vi "ReplaceSelf.vi"(0 "XRef":T13, 1 "Terms":T10, 2 "Diagram":T9, 3 "State In":T4 {"BlockNodeState"."Draw Style" items=["FunctionBlock", "ExpressVI", "Variable", "Elemental I/O", "32x32 Icon", "FunctionBlockCompact"]; "BlockNodeState"."Terminal Data"."Terminal Flags" format="%.0b"}) -> (14 "Replace Self?":T3, 15 "Reply":T1)   [LabVIEW 2018, in "N9010A_SCPI Node.xnode"]
uses:
  N9010A_SCPI Node.xnode
  <vilib>/XNodeSupport/XNodeXNodeRef.ctl
  <vilib>/XNodeSupport/XNodeTermIDPairs.ctl
  <vilib>/XNodeSupport/XNodeTermIDPair.ctl
  <vilib>/XNodeSupport/XNodeTermRef.ctl
  <vilib>/XNodeSupport/XNodeString.ctl
  <vilib>/XNodeSupport/XNodeTopLevelDiagramRef.ctl
  State.ctl
  <vilib>/BlockNodeSupport/BlockNodeState.ctl
  <vilib>/BlockNodeSupport/TerminalData.ctl
  <vilib>/picture/picture.llb/imagedata.ctl
  Utility/command_spec.ctl
  <vilib>/XNodeSupport/XNodeBool.ctl
  <vilib>/XNodeSupport/XNodeStringArray.ctl
  <vilib>/Utility/miscctls.llb/LVPointTypeDef.ctl
  <vilib>/XNodeSupport/NI_XNodeSupport.lvlib
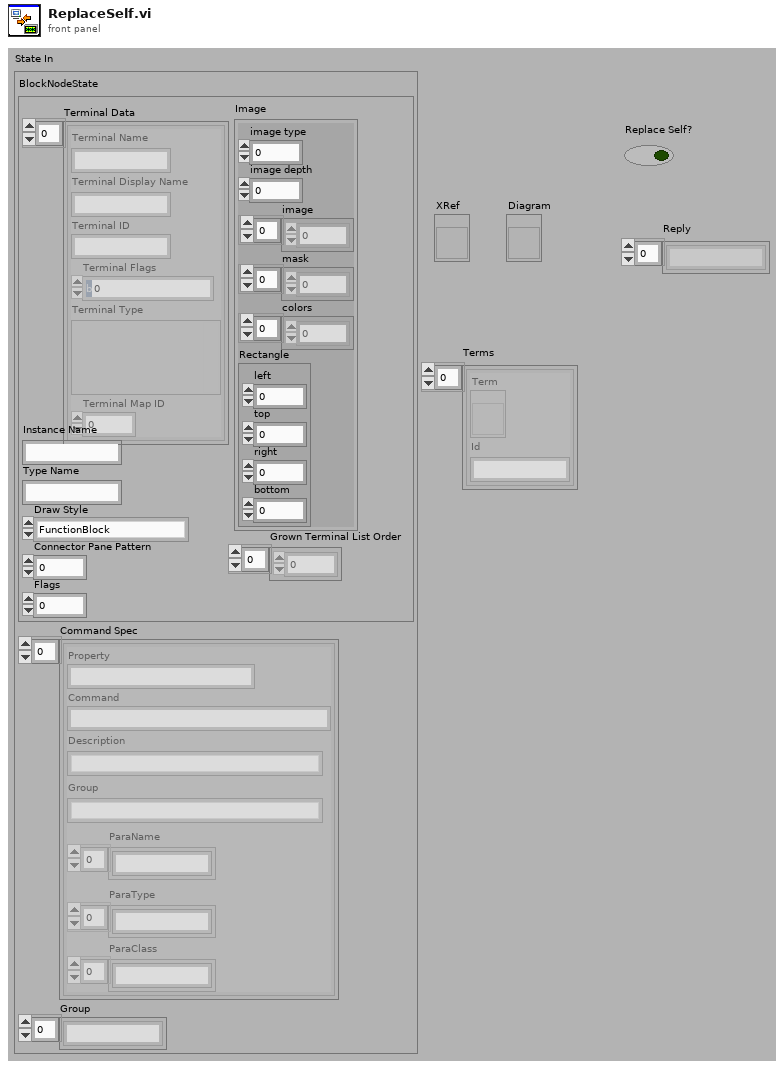
[diagram p1: front panel]
types:
  T1 = typedef "NI_XNodeSupport.lvlib/XNodeStringArray.ctl" = T2[]
  T2 = typedef "NI_XNodeSupport.lvlib/XNodeString.ctl" = string
  T3 = typedef "NI_XNodeSupport.lvlib/XNodeBool.ctl" = bool
  T4 = typedef "N9010A_SCPI Node.xnode/State.ctl" = cluster{"BlockNodeState":T5, "Command Spec":T8, "Group":string[]}
  T5 = typedef "BlockNodeState.ctl" = cluster{"Terminal Data":T6[], "Instance Name":string, "Type Name":string, "Draw Style":i32, "Connector Pane Pattern":i32, "Flags":i32, "Grown Terminal List Order":i32[], "Image":T7}
  T6 = typedef "TerminalData.ctl" = cluster{"Terminal Name":string, "Terminal Display Name":string, "Terminal ID":string, "Terminal Flags":i32, "Terminal Type":variant, "Terminal Map ID":i32}
  T7 = typedef "imagedata.ctl" = cluster{"image type":i32, "image depth":i32, "image":u8[], "mask":u8[], "colors":u32[], "Rectangle":cluster{"left":i16, "top":i16, "right":i16, "bottom":i16}}
  T8 = typedef "command_spec.ctl" = cluster{"Property":string, "Command":string, "Description":string, "Group":string, "ParaName":string[], "ParaType":string[], "ParaClass":string[]}[]
  T9 = typedef "NI_XNodeSupport.lvlib/XNodeTopLevelDiagramRef.ctl" = refnum<vi>
  T10 = typedef "NI_XNodeSupport.lvlib/XNodeTermIDPairs.ctl" = T11[]
  T11 = typedef "NI_XNodeSupport.lvlib/XNodeTermIDPair.ctl" = cluster{"Term":T12, "Id":T2}
  T12 = typedef "NI_XNodeSupport.lvlib/XNodeTermRef.ctl" = refnum<vi>
  T13 = typedef "NI_XNodeSupport.lvlib/XNodeXNodeRef.ctl" = refnum<vi>
  T14 = typedef "LVPointTypeDef.ctl" = cluster{"Horizontal":i16, "Vertical":i16}
  T15 = cluster{"Property":string, "Command":string, "Description":string, "Group":string, "ParaName":string[], "ParaType":string[], "ParaClass":string[]}
  T16 = typedef "LVRectTypeDef.ctl" = cluster{"Left":i16, "Top":i16, "Right":i16, "Bottom":i16}
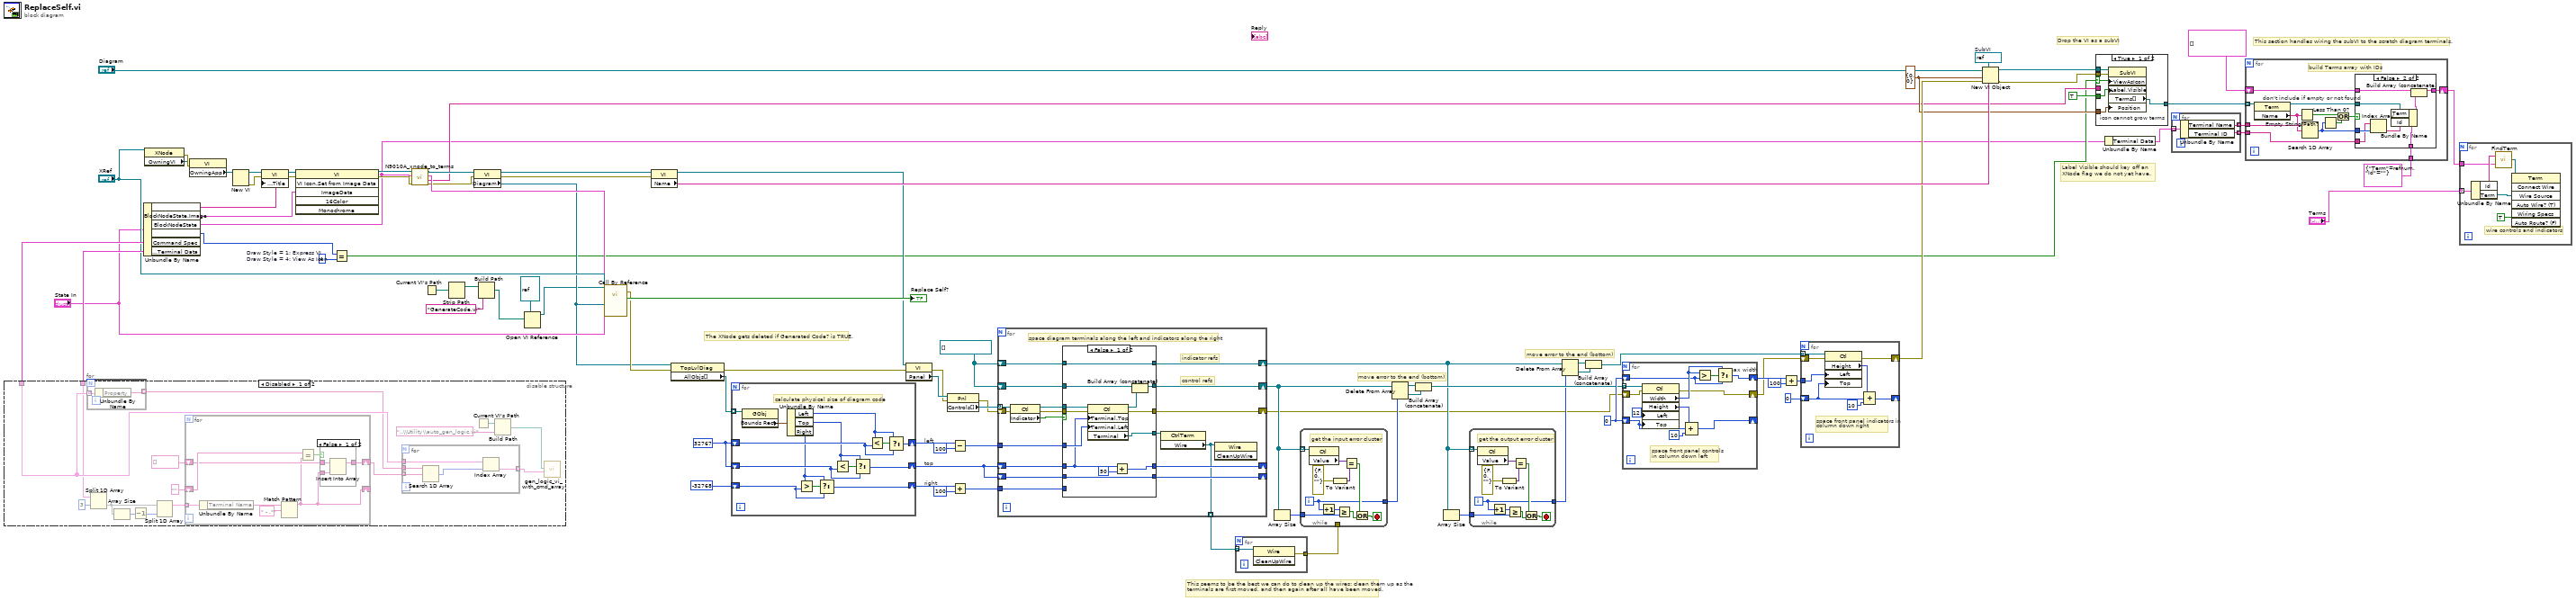
[diagram p0: block diagram]
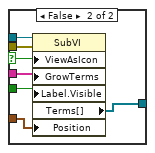
[diagram p2: hidden frame]
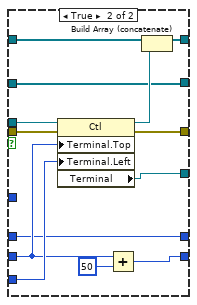
[diagram p4: hidden frame]
diagram:
  w6 = 4  # Draw Style = 1: Express VI Draw Style = 4: View As Icon
  w45 = 0 ("Position:Left")
  w46 = refnum<vi>[] []
  w60 = i16 32767 ("left")
  w8 = T14 {"Horizontal"=0, "Vertical"=0} ("location")
  w79 = refnum<vi> refnum  # SubVI
  # "Label Visible should key off an XNode flag we do not yet have."
  # "Drop the VI as a subVI"
  # "This section handles wiring the subVI to the scratch diagram terminals."
  # "The XNode gets deleted if Generated Code? is TRUE."
  # "This seems to be the best we can do to clean up the wires: clean them up as the terminals are first moved, and then again after all have been moved."
  # "move error to the end (bottom)"
  # "move error to the end (bottom)"
  # "right"
  # "top"
  # "left"
  n1 = Unbundle By Name("State In") -> ("BlockNodeState.Type Name"=w83:string, "BlockNodeState.Image"=w82:T7, "BlockNodeState"=w2:T5, "BlockNodeState.Draw Style"=w5:i32, "Command Spec"=w77:T8, "BlockNodeState.Terminal Data"=w76:T6[])
  n2 = disable-structure shown="Disabled" {
    disable-tunnel: w77 -> [w103 _]
    disable-tunnel: w76 -> [w102 _]
    frame Disabled {
      n3 = for {
        tunnel: [w121] -> _ mode=indexing
        tunnel: [w122] -> w93 mode=indexing
        tunnel: w103 -> [w121] mode=indexing
        n4 = Unbundle By Name(w121) -> ("Property"=w122:string)
      }
      n5 = Split 1D Array(array=w102, index=3) -> (second subarray=w98:T6[])  [unwired: 1 out]
      n6 = Array Size(array=w98) -> (size(s)=w100:i32)
      n7 = Decrement(x=w100) -> (x-1=w99:i32)
      n8 = Split 1D Array(array=w98, index=w99) -> (first subarray=w97:T6[])  [unwired: 1 out]
      n9 = for {
        tunnel: w97 -> [w116] mode=indexing
        shift-right: [w110] -> w94
        shift-left: string[] [] -> [w111]
        shift-right: [w109] -> _
        shift-left: "" ("Terminal Name") -> [w113]
        n10 = Unbundle By Name(w116) -> ("Terminal Name"=w114:string)
        n11 = Match Pattern(string=w114, regular expression=" - .*") -> (before substring=w109:string)  [unwired: 1 in, 3 out]
        n12 = Equal?(x=w113, y=w109) -> (x = y?=w112:bool)
        n13 = case shown="False" w112 {
          tunnel: w111 -> [w119 w120]
          tunnel: w109 -> [w118 _]
          tunnel: [w117 w120] -> w110
          frame False {
            n14 = Insert Into Array(array=w119, new element=w118) -> (w117:string[])  [unwired: 1 in]
          }
          frame True {
          }
        }
      }
      n15 = for {
        tunnel: [w107] -> w92 mode=indexing
        tunnel: w103 -> [w106]
        tunnel: w93 -> [w105]
        tunnel: w94 -> [w104] mode=indexing
        n16 = Search 1D Array(1D array=w105, element=w104) -> (index of element=w108:i32)  [unwired: 1 in]
        n17 = Index Array(array=w106, index=w108) -> (element=w107:T15)
      }
      n18 = Current VI's Path() -> (path=w90:path)
      n19 = Build Path(base path=w90, name or relative path="..\\Utility\\auto_gen_logic.vi") -> (appended path=w89:path)
      n20 = call "gen_logic_vi_with_cmd_array.vi"("CmdInfo"=w92, "VI Paths"=w89) -> ()  [unwired: 9 in, 1 out]
    }
    frame Enabled {
    }
  }
  n21 = property class="XNode"(reference="XRef") -> (error out=w87:errorcluster, "OwningVI"=w86:refnum<vi>)  [unwired: 1 in, 1 out]
  n22 = property class="VI"(reference=w86, error in=w87) -> ("OwningApp"=w88:refnum<vi>)  [unwired: 2 out]
  n23 = New VI(11:w88) -> (0:w85:errorcluster, 3:w84:refnum<vi>)  [unwired: 1 in, 5 out]
  n24 = property class="VI"(reference=w84, error in=w85, "Front Panel.Title"=w83) -> (reference out=w80:refnum<vi>, error out=w81:errorcluster)
  n25 = invoke class="VI" method="VI Icon.Set from Image Data"(reference=w80, error in=w81, "ImageData"=w82) -> (reference out=w63:refnum<vi>, error out=w64:errorcluster)  [unwired: 3 in, 4 out]
  n26 = Equal?(x=w5, y=w6) -> (x = y?=w4:bool)
  n27 = call "N9010A_xnode_to_terms.vi"("error in (no error)"=w64, "BlockNodeState"=w2, "VI Refnum"=w63) -> ("error out"=w19:errorcluster, "GrownTerms"=w7:string[], "Terms"=w62:T10, "VI Refnum out"=w65:refnum<vi>)  [unwired: 5 in]
  n28 = Current VI's Path() -> (path=w71:path)
  n29 = Strip Path(path=w71) -> (stripped path=w72:path)  [unwired: 1 out]
  n30 = property class="VI"(reference=w65, error in=w19) -> (reference out=w75:refnum<vi>, error out=w20:errorcluster, "Diagram"=w26:refnum<vi>)
  n31 = Build Path(base path=w72, name or relative path="GenerateCode.vi") -> (appended path=w69:path)
  n32 = Open VI Reference(type specifier VI Refnum (for type only)=refnum<vi> refnum, vi path=w69) -> (vi reference=w1:refnum<vi>)  [unwired: 2 in, 3 out]
  n33 = call-by-ref "?"(reference=w1, "XRef"="XRef", "Terms"=w62, "Diagram"=w26, "State In"="State In") -> (error out=w27:errorcluster, "Generated Code?"=→"Replace Self?":T3)  [unwired: 14 in, 3 out]
  n34 = property class="VI"(reference=w75, error in=w20) -> (reference out=w25:refnum<vi>, "Name"=w74:string)  [unwired: 1 out]
  n35 = property class="TopLvlDiag"(reference=w26, error in=w27) -> (error out=w51:errorcluster, "AllObjs[]"=w61:refnum<vi>[])  [unwired: 1 out]
  n36 = for {
    tunnel: w61 -> [w136] mode=indexing
    shift-right: [w132] -> w58
    shift-left: w60 -> [w130]
    shift-right: [w133] -> w52
    shift-left: w60 -> [w127]
    shift-right: [w134] -> w54
    shift-left: i16 -32768 ("left") -> [w123]
    # "calculate physical size of diagram code"
    n37 = property class="GObj"(reference=w136) -> ("Bounds Rect"=w135:T16)  [unwired: 1 in, 2 out]
    n38 = Unbundle By Name(w135) -> ("Left"=w124:i16, "Top"=w125:i16, "Right"=w126:i16)
    n39 = Greater?(x=w126, y=w123) -> (0:w128:bool)
    n40 = Select(t=w126, s=w128, f=w123) -> (s? t:f=w134:i16)
    n41 = Less?(x=w125, y=w127) -> (x < y?=w129:bool)
    n42 = Select(t=w125, s=w129, f=w127) -> (s? t:f=w133:i16)
    n43 = Less?(x=w124, y=w130) -> (x < y?=w131:bool)
    n44 = Select(t=w124, s=w131, f=w130) -> (s? t:f=w132:i16)
  }
  n45 = property class="VI"(reference=w25, error in=w51) -> (error out=w48:errorcluster, "Panel"=w50:refnum<vi>)  [unwired: 1 out]
  n46 = property class="Pnl"(reference=w50, error in=w48) -> (error out=w47:errorcluster, "Controls[]"=w49:refnum<vi>[])  [unwired: 1 out]
  n47 = Subtract(x=w58, y=i16 100) -> (x-y=w57:i16)
  n48 = Add(x=w54, y=i16 100) -> (x+y=w53:i16)
  n49 = for {
    tunnel: w57 -> [w149]
    tunnel: w53 -> [w154]
    shift-right: [w150] -> _
    shift-left: w52 -> [w151]
    shift-right: [w152] -> _
    shift-left: w52 -> [w153]
    tunnel: w49 -> [w146] mode=indexing
    shift-right: [w144] -> w28
    shift-left: w47 -> [w143]
    shift-right: [w140] -> w35
    shift-left: w46 -> [w141]
    shift-right: [w138] -> w29
    shift-left: w46 -> [w139]
    tunnel: [w137] -> w23 mode=indexing
    # "indicator refs"
    # "control refs"
    # "space diagram terminals along the left and indicators along the right"
    n50 = property class="Ctl"(reference=w146, error in=w143) -> (reference out=w148:refnum<vi>, error out=w145:errorcluster, "Indicator"=w147:bool)
    n51 = case shown="False" w147 {
      tunnel: w148 -> [w167 w180]
      tunnel: w154 -> [_ w179]
      tunnel: w153 -> [w163 w177]
      tunnel: [w163 w176] -> w152
      tunnel: w151 -> [w160 w175]
      tunnel: [w164 w175] -> w150
      tunnel: w149 -> [w165 _]
      tunnel: w145 -> [w161 w174]
      tunnel: [w162 w173] -> w144
      tunnel: [w159 w172] -> w142
      tunnel: w141 -> [w157 w170]
      tunnel: [w156 w170] -> w140
      tunnel: w139 -> [w155 w169]
      tunnel: [w155 w168] -> w138
      frame False {
        n52 = property class="Ctl"(reference=w167, error in=w161, "Terminal.Top"=w160, "Terminal.Left"=w165) -> (reference out=w158:refnum<vi>, error out=w162:errorcluster, "Terminal"=w159:refnum<vi>)
        n53 = Add(x=w160, y=i16 50) -> (x+y=w164:i16)
        n54 = Build Array (concatenate)(w157, w158) -> (w156:refnum<vi>[])
      }
      frame True {
        n55 = property class="Ctl"(reference=w180, error in=w174, "Terminal.Top"=w177, "Terminal.Left"=w179) -> (reference out=w171:refnum<vi>, error out=w173:errorcluster, "Terminal"=w172:refnum<vi>)
        n56 = Add(x=w177, y=i16 50) -> (x+y=w176:i16)
        n57 = Build Array (concatenate)(w169, w171) -> (w168:refnum<vi>[])
      }
    }
    n58 = property class="CtrlTerm"(reference=w142) -> ("Wire"=w137:refnum<vi>)  [unwired: 1 in, 2 out]
    n59 = invoke class="Wire" method="CleanUpWire"(reference=w137) -> ()  [unwired: 2 in, 3 out]
  }
  n60 = for {
    tunnel: w23 -> [w182] mode=indexing
    tunnel: [w181] -> w24
    n61 = invoke class="Wire" method="CleanUpWire"(reference=w182) -> (error out=w181:errorcluster)  [unwired: 2 in, 2 out]
  }
  n62 = Array Size(array=w35) -> (size(s)=w39:i32)
  n63 = while {
    tunnel: w35 -> [w192] mode=indexing
    tunnel: w39 -> [w187]
    tunnel: [w183] -> w38
    tunnel: w24 -> [_]
    i -> [w183]
    stop <- w185 stop-if-true
    # "get the input error cluster"
    n64 = property class="Ctl"(reference=w192) -> ("Value"=w191:variant)  [unwired: 1 in, 2 out]
    n65 = Increment(x=w183) -> (x+1=w184:i32)
    n66 = To Variant(anything=errorcluster {"status"=FALSE, "code"=0, "source"=""} ("error in (no error)")) -> (Variant=w189:variant)
    n67 = Greater Or Equal?(x=w184, y=w187) -> (x >= y?=w186:bool)
    n68 = Equal?(x=w191, y=w189) -> (x = y?=w188:bool)
    n69 = Or(x=w188, y=w186) -> (x .or. y?=w185:bool)
  }
  n70 = Delete From Array(array=w35, index=w38) -> (deleted portion=w36:refnum<vi>, array with subset deleted=w37:refnum<vi>[])  [unwired: 1 in]
  n71 = Build Array (concatenate)(w37, w36) -> (w34:refnum<vi>[])
  n72 = Array Size(array=w29) -> (size(s)=w33:i32)
  n73 = while {
    tunnel: w29 -> [w202] mode=indexing
    tunnel: w33 -> [w197]
    tunnel: [w194] -> w30
    i -> [w194]
    stop <- w195 stop-if-true
    # "get the output error cluster"
    n74 = property class="Ctl"(reference=w202) -> ("Value"=w201:variant)  [unwired: 1 in, 2 out]
    n75 = Increment(x=w194) -> (x+1=w193:i32)
    n76 = To Variant(anything=errorcluster {"status"=FALSE, "code"=0, "source"=""} ("error in (no error)")) -> (Variant=w199:variant)
    n77 = Greater Or Equal?(x=w193, y=w197) -> (x >= y?=w196:bool)
    n78 = Equal?(x=w201, y=w199) -> (x = y?=w198:bool)
    n79 = Or(x=w198, y=w196) -> (x .or. y?=w195:bool)
  }
  n80 = Delete From Array(array=w29, index=w30) -> (deleted portion=w32:refnum<vi>, array with subset deleted=w31:refnum<vi>[])  [unwired: 1 in]
  n81 = Build Array (concatenate)(w31, w32) -> (w22:refnum<vi>[])
  n82 = for {
    tunnel: w34 -> [w214] mode=indexing
    shift-right: [w209] -> _
    shift-left: w45 -> [w211]
    shift-right: [w205] -> w43
    shift-left: w45 -> [w206]
    shift-right: [w203] -> w41
    shift-left: w28 -> [w204]
    # "space front panel controls in column down left"
    # "max width"
    n83 = property class="Ctl"(reference=w214, error in=w204, "Left"=12 ("Position:Left"), "Top"=w211) -> (error out=w203:errorcluster, "Width"=w207:u32, "Height"=w212:u32)  [unwired: 1 out]
    n84 = Compound Arithmetic op=ADD(w212, w211, 10 ("value")) -> (w209:u32)
    n85 = Greater?(x=w207, y=w206) -> (0:w208:bool)
    n86 = Select(t=w207, s=w208, f=w206) -> (s? t:f=w205:u32)
  }
  n87 = Add(x=w43, y=u32 100) -> (x+y=w42:u32)
  n88 = for {
    tunnel: w22 -> [w222] mode=indexing
    tunnel: w42 -> [w221]
    shift-right: [w219] -> w21
    shift-left: w41 -> [w220]
    shift-right: [w215] -> _
    shift-left: 0 ("Position:Left") -> [w216]
    # "space front panel indicators in column down right"
    n89 = property class="Ctl"(reference=w222, error in=w220, "Left"=w221, "Top"=w216) -> (error out=w219:errorcluster, "Height"=w217:u32)  [unwired: 1 out]
    n90 = Compound Arithmetic op=ADD(w217, w216, 10 ("value")) -> (w215:u32)
  }
  n91 = New VI Object(vi object class=w79, owner refnum="Diagram", position/next to=w8, 6:w74, 8:w21) -> (object refnum=w10:refnum<vi>, 0:w9:errorcluster)  [unwired: 3 out]
  n92 = case shown="True" w4 {
    selector: w4 -> [w223 w229]
    tunnel: [w228 w235] -> w13
    tunnel: TRUE ("Label.Visible") -> [w227 w234]
    tunnel: w10 -> [w226 w233]
    tunnel: w8 -> [w225 w232]
    tunnel: w7 -> [_ w231]
    tunnel: w9 -> [w224 w230]
    frame True {
      # "icon cannot grow terms"
      n93 = property class="SubVI"(reference=w226, error in=w224, "ViewAsIcon"=w223, "Label.Visible"=w227, "Position"=w225) -> ("Terms[]"=w228:refnum<vi>[])  [unwired: 2 out]
    }
    frame False {
      n94 = property class="SubVI"(reference=w233, error in=w230, "ViewAsIcon"=w229, "GrowTerms"=w231, "Label.Visible"=w234, "Position"=w232) -> ("Terms[]"=w235:refnum<vi>[])  [unwired: 2 out]
    }
  }
  n95 = Unbundle By Name(w2) -> ("Terminal Data"=w12:T6[])
  n96 = for {
    tunnel: w12 -> [w238] mode=indexing
    tunnel: [w237] -> w14 mode=indexing
    tunnel: [w236] -> w15 mode=indexing
    n97 = Unbundle By Name(w238) -> ("Terminal Name"=w237:string, "Terminal ID"=w236:string)
  }
  n98 = for {
    tunnel: w13 -> [w250] mode=indexing
    tunnel: w14 -> [w249]
    tunnel: w15 -> [w240]
    tunnel: T11 {"Term"=refnum, "Id"=""} ("Code Gen Term") -> [w247]
    shift-right: [w245] -> w18
    shift-left: T11[] [] -> [w246]
    # "don't include if empty or not found"
    # "build Terms array with IDs"
    n99 = property class="Term"(reference=w250) -> (reference out=w248:refnum<vi>, "Name"=w239:string)  [unwired: 1 in, 1 out]
    n100 = Empty String/Path?(string/path=w239) -> (empty?=w244:bool)
    n101 = Search 1D Array(1D array=w249, element=w239) -> (index of element=w243:i32)  [unwired: 1 out]
    n102 = Less Than 0?(x=w243) -> (x < 0?=w241:bool)
    n103 = Or(x=w244, y=w241) -> (x .or. y?=w242:bool)
    n104 = case shown="False" w242 {
      tunnel: w248 -> [_ w259]
      tunnel: w247 -> [_ w256]
      tunnel: w246 -> [w251 w255]
      tunnel: [w251 w254] -> w245
      tunnel: w243 -> [_ w253]
      tunnel: w240 -> [_ w252]
      frame True {
      }
      frame False {
        n105 = Index Array(array=w252, index=w253) -> (element=w258:string)
        n106 = Bundle By Name(cluster=w256, "Term"=w259, "Id"=w258) -> (w257:T11)
        n107 = Build Array (concatenate)(w255, w257) -> (w254:T11[])
      }
    }
  }
  n108 = for {
    tunnel: "Terms" -> [w264] mode=indexing
    tunnel: w18 -> [w261]
    # "wire controls and indicators"
    n109 = Unbundle By Name(w264) -> ("Id"=w262:T2, "Term"=w263:T12)
    n110 = call <vilib>:"FindTerm.vi"("Terms"=w261, "String"=w262) -> ("Term"=w260:refnum<vi>)
    n111 = invoke class="Term" method="Connect Wire"(reference=w260, "Wire Source"=w263, "Auto Route? (F)"=TRUE) -> ()  [unwired: 4 in, 7 out]
  }
